vi "Update Time.vi"(8 "error in (no error)":errorcluster, 11 "Time in":i64) -> (0 "error out":errorcluster, 3 "Time out":i64)   [LabVIEW 2021, in "ChannelCommon.lvlib"]
uses:
  ChannelCommon.lvlib
  <vilib>/CIF Foundation/CIF Utilities/Time/System Time/LabVIEW Time to TAI Time.vi
  <vilib>/CIF Foundation/CIF Utilities/Time/Time_CIF_U.lvlib
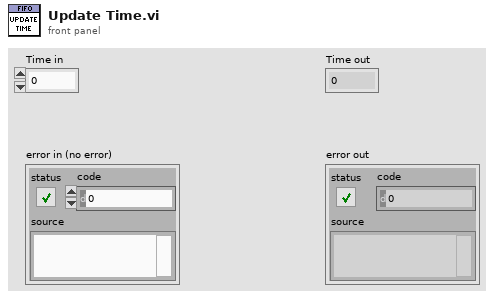
[diagram p1: front panel]
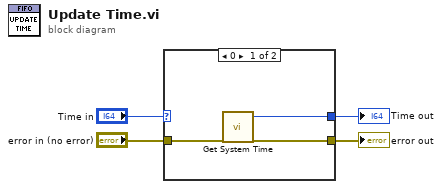
[diagram p0: block diagram]
diagram:
  n1 = case shown="0" "Time in" {
    selector: "Time in" -> [_ w8]
    tunnel: [w6 w8] -> w3
    tunnel: "error in (no error)" -> [w5 w7]
    tunnel: [w5 w7] -> w1
    frame 0 {
      n2 = call <vilib>:"Get System Time.vi"() -> ("Time (ns)"=w6:i64)  [unwired: 5 in]
    }
    frame 1, Default {
    }
  }
  "Time out" <- w3
  "error out" <- w1
